vi "TCP Client  单向通信.vi"() -> ()   [LabVIEW 2015]
panel:
  in  "Waveform":waveform(dbl)
  in  "stop":bool
  out "Waveform Graph":waveform(dbl)(graph)
  in  "remote port or service name":u16
  in  "address":string
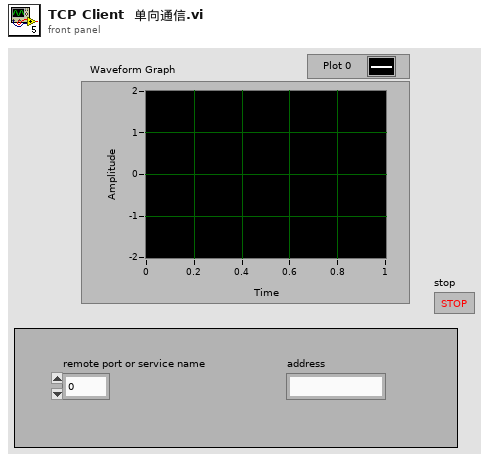
[diagram p1: front panel]
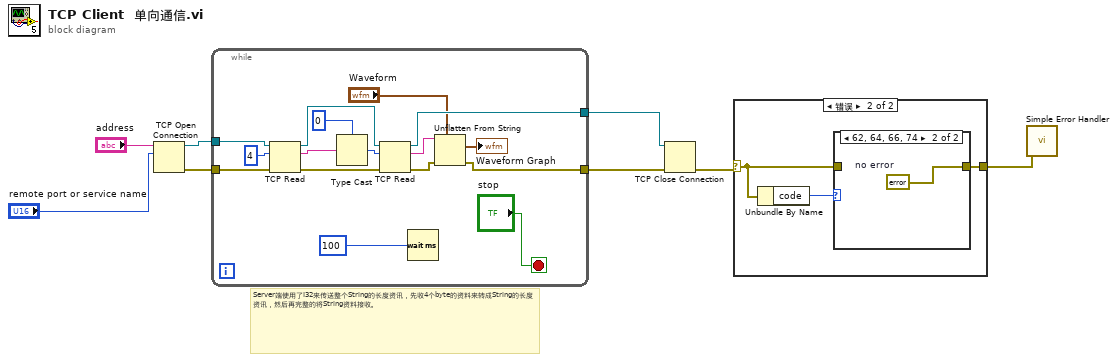
[diagram p0: block diagram]
diagram:
  # "Server端使用了I32来传送整个String的长度资讯，先收4个byte的资料来转成String的长度资讯，然后再完整的将String资料接收。"
  n1 = TCP Open Connection(address="address", remote port or service name="remote port or service name") -> (connection ID=w6:refnum<k5>, error out=w5:errorcluster)  [unwired: 3 in]
  n2 = while {
    tunnel: w6 -> [w16]
    tunnel: w5 -> [w14]
    tunnel: [w13] -> w4
    tunnel: [w9] -> w3
    stop <- "stop" stop-if-true
    n3 = TCP Read(connection ID=w16, bytes to read=4, error in (no error)=w14) -> (connection ID out=w24:refnum<k5>, data out=w22:string, error out=w23:errorcluster)  [unwired: 2 in]
    n4 = Type Cast(type=0, x=w22) -> (*(type *) &x=w21:i32)
    n5 = TCP Read(connection ID=w24, bytes to read=w21, error in (no error)=w23) -> (connection ID out=w13:refnum<k5>, data out=w12:string, error out=w10:errorcluster)  [unwired: 2 in]
    n6 = Wait (ms)(milliseconds to wait=u32 100) -> ()  [unwired: 1 out]
    n7 = Unflatten From String(type="Waveform", binary string=w12, error in (no error)=w10) -> (value=→"Waveform Graph":waveform(dbl), error out=w9:errorcluster)  [unwired: 2 in, 1 out]
  }
  n8 = TCP Close Connection(connection ID=w4, error in (no error)=w3) -> (error out=w1:errorcluster)  [unwired: 1 in, 1 out]
  n9 = case shown="错误" w1 {
    selector: w1 -> [w25 w27]
    tunnel: [w25 w28] -> w2
    frame No Error {
    }
    frame Error {
      n10 = Unbundle By Name(w27) -> ("code"=w26:i32)
      n11 = case shown="62, 64, 66, 74" w26 {
        tunnel: [w29 w30] -> w28
        tunnel: w27 -> [w29 _]
        frame Default {
        }
        frame 62, 64, 66, 74 {
          w30 = errorcluster {"status"=FALSE, "code"=0, "source"=""}  # no error
        }
      }
    }
  }
  n12 = call <vilib>:"Simple Error Handler.vi"("error in (no error)"=w2) -> ()  [unwired: 4 in, 5 out]
